vi "Write VRef.vi"(8 "error in (no error)":errorcluster, 10 "VRef (5V)":dbl=5.0, 11 "LINX-DAC8552 in":refnum<class "LINX-DAC8552.lvclass">) -> (0 "error out":errorcluster, 3 "LINX-DAC8552 out":refnum<class "LINX-DAC8552.lvclass">)   [LabVIEW 2020, in "LINX-DAC8552.lvclass"]
uses:
  LINX-DAC8552.lvclass
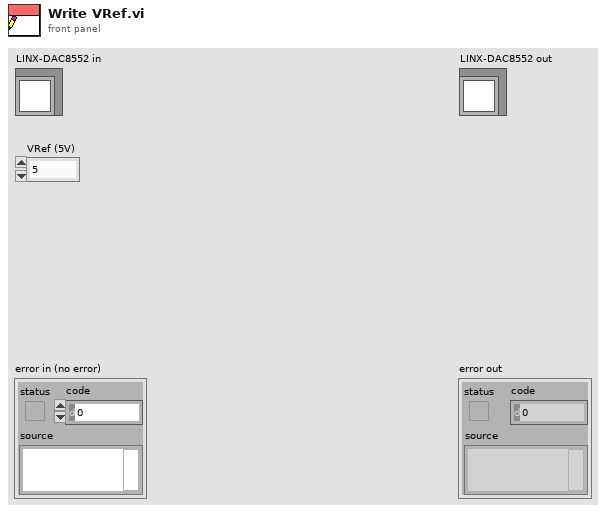
[diagram p1: front panel]
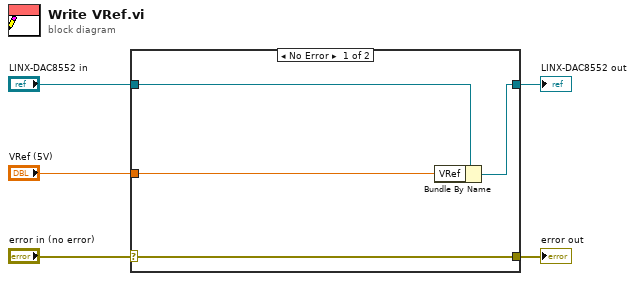
[diagram p0: block diagram]
diagram:
  n1 = case shown="No Error" "error in (no error)" {
    selector: "error in (no error)" -> [w9 w10]
    tunnel: [w9 w10] -> w4
    tunnel: [w7 w11] -> w2
    tunnel: "LINX-DAC8552 in" -> [w8 w11]
    tunnel: "VRef (5V)" -> [w6 _]
    frame No Error {
      n2 = Bundle By Name(cluster=w8, "VRef"=w6) -> (w7:refnum<class "LINX-DAC8552.lvclass">)
    }
    frame Error {
    }
  }
  "error out" <- w4
  "LINX-DAC8552 out" <- w2
